vi "DataLog Delete Tag Log Directory.vi"(0 "tag log directory":path, 11 "error in (no error)":errorcluster) -> (4 "dup tag log directory":path, 15 "error out":errorcluster)   [LabVIEW 2012]
doc: "Deletes a tag log directory after deleting any files contained therein. If the log directory contains one or more subdirectories (which typically belong to the log of a meta tag) an error is returned."
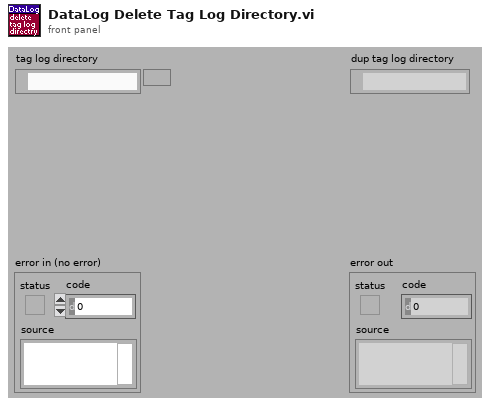
[diagram p1: front panel]
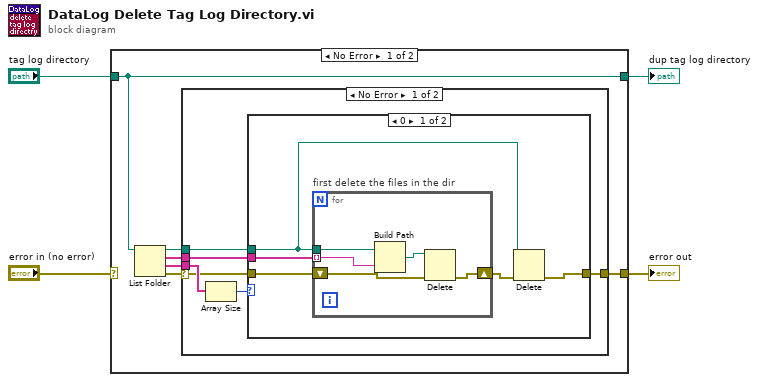
[diagram p0: block diagram]
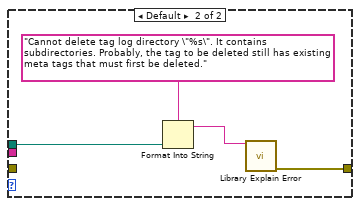
[diagram p2: hidden frame]
diagram:
  n1 = case shown="No Error" "error in (no error)" {
    selector: "error in (no error)" -> [_ w33]
    tunnel: [w8 w33] -> w4
    tunnel: "tag log directory" -> [w10 w32]
    tunnel: [w10 w32] -> w1
    frame No Error {
      n2 = List Folder(path=w10) -> (path out=w5:path, filenames=w7:string[], folder names=w6:string[], error out=w9:errorcluster)  [unwired: 3 in]
      n3 = case shown="No Error" w9 {
        selector: w9 -> [w12 w31]
        tunnel: [w14 w31] -> w8
        tunnel: w7 -> [w11 _]
        tunnel: w6 -> [w16 _]
        tunnel: w5 -> [w13 _]
        frame No Error {
          n4 = Array Size(array=w16) -> (size(s)=w15:i32)
          n5 = case shown="0" w15 {
            tunnel: [w17 w30] -> w14
            tunnel: w13 -> [w18 w29]
            tunnel: w12 -> [w21 _]
            tunnel: w11 -> [w20 _]
            frame 0 {
              n6 = for "first delete the files in the dir" {
                shift-right: [w22] -> w19
                shift-left: w21 -> [w24]
                tunnel: w18 -> [w26]
                tunnel: w20 -> [w25] mode=indexing
                n7 = Build Path(base path=w26, name or relative path=w25) -> (appended path=w23:path)
                n8 = Delete(path (use dialog)=w23, error in=w24) -> (error out=w22:errorcluster)  [unwired: 3 in, 2 out]
              }
              n9 = Delete(path (use dialog)=w18, error in=w19) -> (error out=w17:errorcluster)  [unwired: 3 in, 2 out]
            }
            frame Default {
              n10 = Format Into String(format string="Cannot delete tag log directory \"%s\". It contains subdirectories. Probably, the tag to be deleted still has existing meta tags that must first be deleted.", w29) -> (resulting string=w27:string)  [unwired: 2 in, 1 out]
              n11 = call "Library Explain Error.vi"("explanation prefix (none)"=w27) -> ("explained error"=w30:errorcluster)  [unwired: 14 in]
            }
          }
        }
        frame Error {
        }
      }
    }
    frame Error {
    }
  }
  "error out" <- w4
  "dup tag log directory" <- w1
